vi "GetPartsinPartStudio.vi"(8 "error in":errorcluster, 11 "Device In":T2) -> (0 "error out":errorcluster, 1 "micro and ID":T1(array[cluster]), 2 "Comm":T3, 3 "Device Out":T2)   [LabVIEW 2019]
uses:
  <userlib>/IoT Devices/_subVIs/HTTPComm.ctl
  <userlib>/Onshape/_SubVI/Cluster.ctl
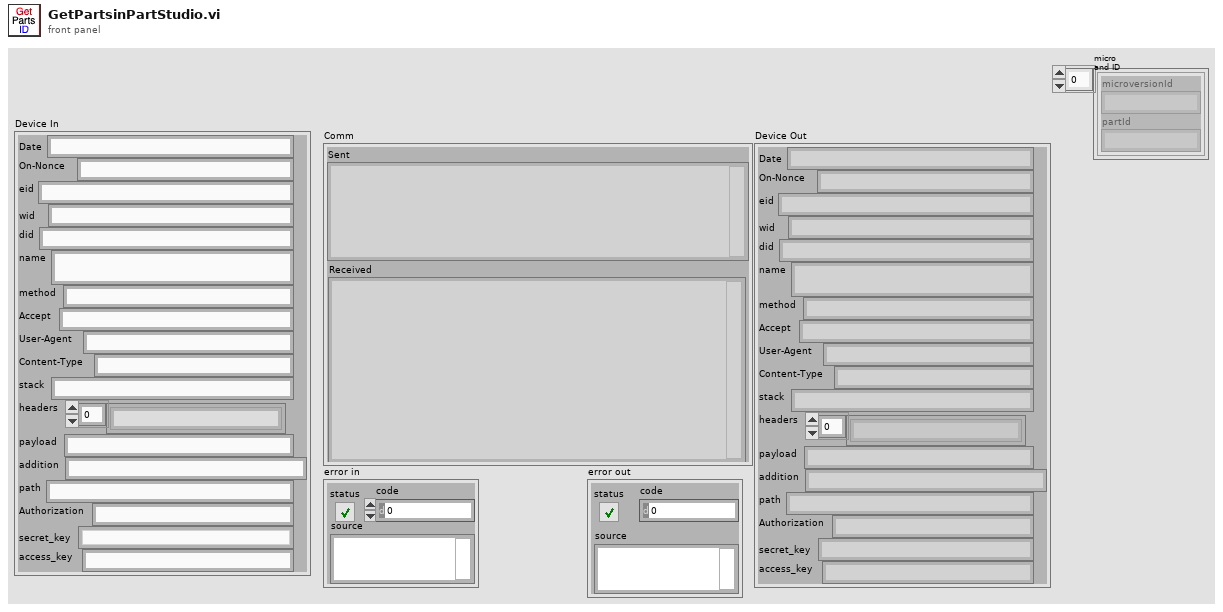
[diagram p1: front panel]
types:
  T1 = cluster{"microversionId":string, "partId":string}[]
  T2 = typedef "Cluster.ctl" = cluster{"Date":string, "On-Nonce":string, "eid":string, "wid":string, "did":string, "name":string, "method":string, "Accept":string, "User-Agent":string, "Content-Type":string, "stack":string, "headers":string[], "payload":string, "addition":string, "path":string, "Authorization":string, "secret_key":string, "access_key":string}
  T3 = typedef "HTTPComm.ctl" = cluster{"url":string, "sent headers":string, "sent body":string, "headers":string, "body":string, "Sent":string, "Received":string}
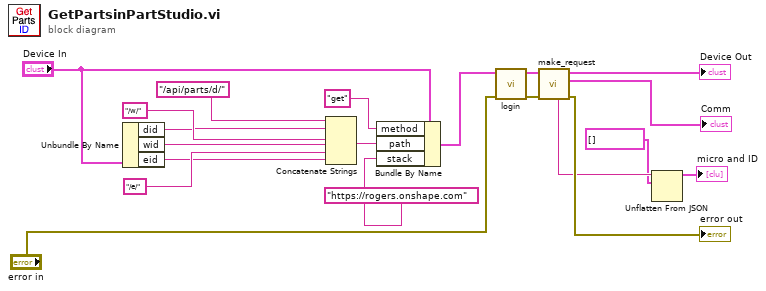
[diagram p0: block diagram]
diagram:
  n1 = Unbundle By Name("Device In") -> ("did"=w9:string, "wid"=w8:string, "eid"=w7:string)
  n2 = Concatenate Strings("/api/parts/d/" ("payload"), w9, "/w/" ("string"), w8, "/e/" ("string"), w7) -> (w16:string)
  n3 = Bundle By Name(cluster="Device In", "method"="get" ("Method"), "path"=w16, "stack"="https://rogers.onshape.com" ("stacks")) -> (w4:T2)
  n4 = call <userlib>:"login.vi"("error in"="error in", "Device In"=w4) -> ("error out"=w11:errorcluster, "Device Out"=w14:T2)  [unwired: 8 in]
  n5 = call <userlib>:"make_request.vi"("Error in"=w11, "Device In"=w14) -> ("error out"=→"error out":errorcluster, "Comm"=→"Comm":T3, "Device Out"=→"Device Out":T2, "body"=w3:string)  [unwired: 5 in, 1 out]
  n6 = Unflatten From JSON(JSON string=w3, type and defaults=T1 []) -> (value=→"micro and ID":T1)  [unwired: 5 in, 1 out]
